vi "AddFailure_FailureMessageSet.vi"() -> (0 "error out":errorcluster)   [LabVIEW 2017, in "ResultTreeListenerTest.lvlib"]
uses:
  ResultTreeListenerTest.lvlib
  ResultTreeListener/ResultTreeListener.lvclass
  ResultTree/ResultTree.lvclass
  Support/FakeTestCase/FakeTestCase.lvclass
  C:/Users/de200256/Code/neuperger/lvunit/Test/Test.lvclass
  275d98eb-69a7-4435-8809-2af3ffd1cf1d.vi
panel:
  in  "Tree":string(tree)
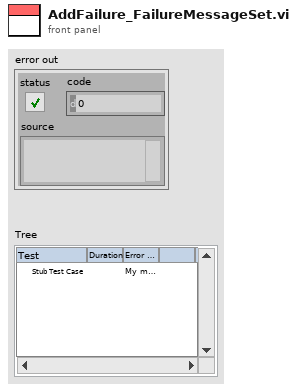
[diagram p1: front panel]
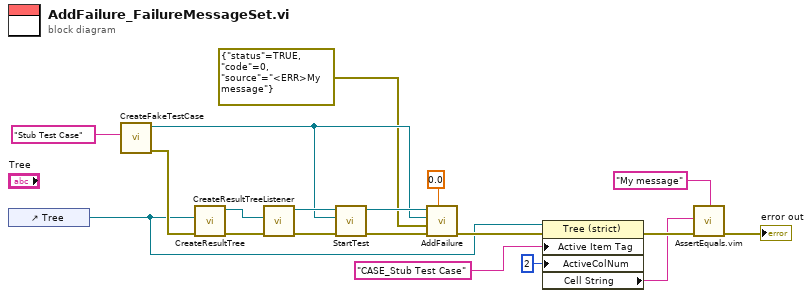
[diagram p0: block diagram]
diagram:
  n1 = control-ref of="Tree"() -> (w6:refnum<vi>)
  n2 = call "CreateFakeTestCase.vi"("Name"="Stub Test Case") -> ("error out"=w11:errorcluster, "FakeTestCase out"=w9:refnum<class "FakeTestCase.lvclass">)  [unwired: 9 in]
  n3 = call "CreateResultTree.vi"("error in (no error)"=w11, "Tree Refnum"=w6) -> ("error out"=w19:errorcluster, "ResultTree out"=w18:refnum<class "ResultTree.lvclass">)  [unwired: 8 in]
  n4 = call "CreateResultTreeListener.vi"("error in (no error)"=w19, "ResultTree"=w18) -> ("error out"=w17:errorcluster, "ResultTreeListener out"=w15:refnum<class "ResultTreeListener.lvclass">)  [unwired: 8 in]
  n5 = call-dynamic "StartTest.vi"("error in (no error)"=w17, "Test"=w9, "ResultTreeListener in"=w15) -> ("error out"=w13:errorcluster, "ResultTreeListener out"=w12:refnum<class "ResultTreeListener.lvclass">)  [unwired: 7 in]
  n6 = call-dynamic "AddFailure.vi"("Time"=0.0, "error in (no error)"=w13, "Failure"=errorcluster {"status"=TRUE, "code"=0, "source"="<ERR>My message"}, "Test"=w9, "ResultTreeListener in"=w12) -> ("error out"=w10:errorcluster)  [unwired: 5 in, 1 out]
  n7 = property class="Tree (strict)"(reference=w6, error in=w10, "Active Item Tag"="CASE_Stub Test Case" ("Active Item:Tag"), "ActiveColNum"=2 ("Active Cell:Active Column Number")) -> (error out=w7:errorcluster, "Cell String"=w2:string)  [unwired: 1 out]
  n8 = call "AssertEquals.vim"("Expected"="My message", "error in (no error)"=w7, "Actual"=w2) -> ("error out"=→"error out":errorcluster)  [unwired: 8 in]
